vi "Initialize.vi"(8 "error in":errorcluster, 11 "FPGA resource name":T2) -> (0 "error out":errorcluster, 3 "FPGA VI Reference Out":T1)   [LabVIEW 2024, in "FPGA Interface.lvlib"]
uses:
  FPGA Interface.lvlib
  <vilib>/userDefined/High Color/nirio_resource_hc.ctl
  Type Definitions/ECU FPGA Reference.ctl
  FPGA Reference - Open.vi
  FPGA Reference - Get.vi
  <vilib>/FPGAPlugInAG/cRIO-9030/niLvFpga_Reset_cRIO-9030.vi
  <vilib>/FPGAPlugInAG/cRIO-9030/niLvFpga_Run_cRIO-9030.vi
  <vilib>/rvi/interface/nirviMethod/nirviMethod.xnode
  FPGA Bitfiles/ecu-9030_FPGATarget_FPGAMain_pDLqQGhG1UY.lvbitx
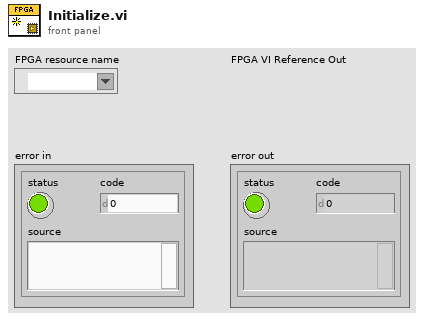
[diagram p1: front panel]
types:
  T1 = typedef "ECU FPGA Reference.ctl" = refnum<k20>
  T2 = typedef "nirio_resource_hc.ctl" = tag
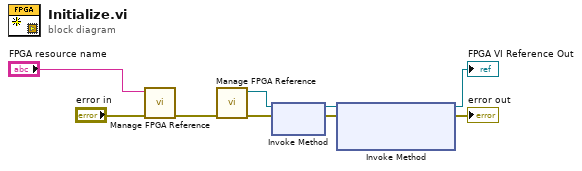
[diagram p0: block diagram]
diagram:
  n1 = call-poly "Manage FPGA Reference.vi"("error in"="error in", "FPGA resource name"="FPGA resource name") -> ("error out"=w3:errorcluster)  [unwired: 9 in]
  n2 = call-poly "Manage FPGA Reference.vi"("error in"=w3) -> ("error out"=w2:errorcluster, "FPGA Reference Out"=w1:T1)  [unwired: 9 in]
  n3 = xnode "Invoke Method"("FPGA VI Reference In"=w1, "error in"=w2) -> ("FPGA VI Reference Out"=w9:T1, "error out"=w8:errorcluster)
  n4 = xnode "Invoke Method"("FPGA VI Reference In"=w9, "error in"=w8) -> ("FPGA VI Reference Out"=→"FPGA VI Reference Out":T1, "error out"=→"error out":errorcluster)  [unwired: 1 in]
